vi "Set Output.vi"(8 "error in (no error)":errorcluster, 10 "Output value":refnum<class "Mag Lab Result.lvclass">, 11 "Visa instrument in":refnum<class "Visa instrument.lvclass">) -> (0 "error out":errorcluster, 2 "Actual output value":refnum<class "Mag Lab Result.lvclass">, 3 "Visa instrument out":refnum<class "Visa instrument.lvclass">)   [LabVIEW 2015, in "Visa instrument.lvclass"]
uses:
  Visa instrument.lvclass
  Mag Lab Result/Mag Lab Result.lvclass
  Mag Lab Hardware.lvclass/Mag Lab Hardware.ctl
  Mag Lab Root/Mag Lab Root.lvclass/Mag Lab Root.ctl
  Mag Lab Error Handler/Mag Lab Error Handler.lvclass
  Mag Lab Hardware.lvclass
  Mag Lab Root/Mag Lab Root.lvclass
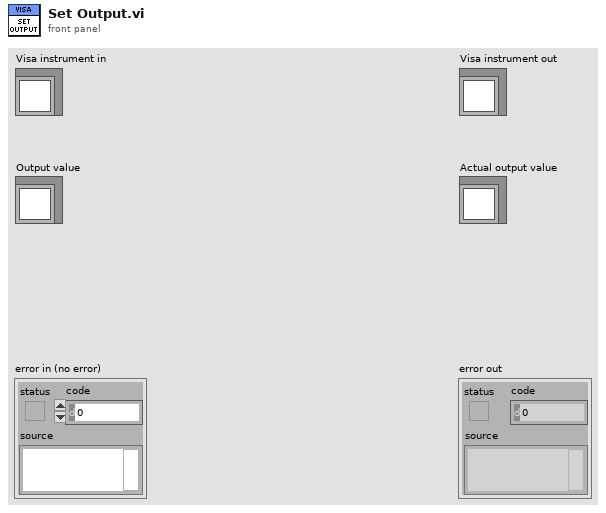
[diagram p1: front panel]
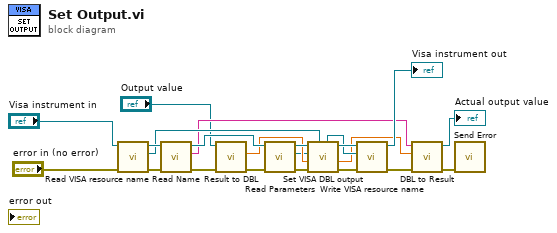
[diagram p0: block diagram]
diagram:
  n1 = call "Read VISA resource name.vi"("error in (no error)"="error in (no error)", "Mag Lab Hardware in"="Visa instrument in") -> ("error out"=w21:errorcluster, "VISA resource name"=w11:refnum<visa-resource-name>, "Mag Lab Hardware out"=w22:refnum<class "Visa instrument.lvclass">)  [unwired: 7 in]
  n2 = call "Read Name.vi"("error in (no error)"=w21, "Mag Lab Root in"=w22) -> ("error out"=w3:errorcluster, "Name"=w7:string, "Mag Lab Root out"=w19:refnum<class "Visa instrument.lvclass">)  [unwired: 7 in]
  n3 = call "Result to DBL.vi"("error in (no error)"=w3, "Mag Lab Result"="Output value") -> ("error out"=w2:errorcluster, "Value"=w4:dbl)  [unwired: 7 in, 1 out]
  n4 = call-dynamic "Read Parameters.vi"("error in (no error)"=w2, "Mag Lab Root in"=w19) -> ("error out"=w15:errorcluster, "Mag Lab Parameters.lvclass"=w1:refnum<class "Mag Lab Parameters.lvclass">, "Mag Lab Root out"=w18:refnum<class "Visa instrument.lvclass">)  [unwired: 7 in]
  n5 = call-dynamic "Set VISA DBL output.vi"("VISA resource name"=w11, "error in (no error)"=w15, "Output value"=w4, "Mag Lab Parameters in"=w1, "Visa instrument in"=w18) -> ("error out"=w16:errorcluster, "Actula output value"=w8:dbl, "Visa instrument out"=w17:refnum<class "Visa instrument.lvclass">, "VISA resource name out"=w10:refnum<visa-resource-name>)  [unwired: 3 in]
  n6 = call "Write VISA resource name.vi"("error in (no error)"=w16, "VISA resource name"=w10, "Mag Lab Hardware in"=w17) -> ("error out"=w20:errorcluster, "Mag Lab Hardware out"=→"Visa instrument out":refnum<class "Visa instrument.lvclass">)  [unwired: 7 in]
  n7 = call "DBL to Result.vi"("error in (no error)"=w20, "Data"=w8, "Name"=w7) -> ("error out"=w14:errorcluster, "Mag Lab Result out"=→"Actual output value":refnum<class "Mag Lab Result.lvclass">)  [unwired: 7 in]
  n8 = call "Send Error.vi"("error in (no error)"=w14) -> ()  [unwired: 9 in, 2 out]
